vi "CheckNextState.vi"(0 "Car Wash IN":T1, 1 "Wash Options":bool[](array[boolean]), 2 "Current Step":i8, 3 "TimeHasElapsed?":bool) -> (7 "Car Wash OUT":T1, 8 "Next Step":i8)   [LabVIEW 2019]
uses:
  Controls/Car Wash Indicators.ctl
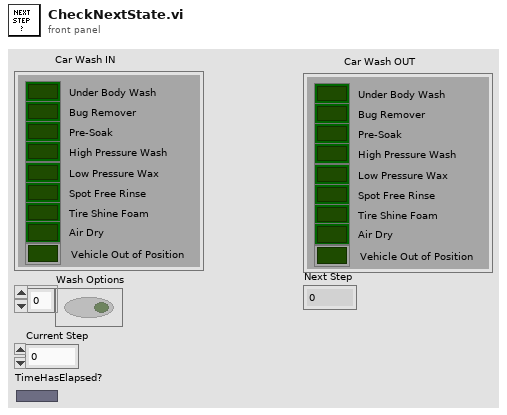
[diagram p1: front panel]
types:
  T1 = typedef "Car Wash Indicators.ctl" = cluster{"Under Body Wash":bool, "Bug Remover":bool, "Pre-Soak":bool, "High Pressure Wash":bool, "Low Pressure Wax":bool, "Spot Free Rinse":bool, "Tire Shine Foam":bool, "Air Dry":bool, "Vehicle Out of Position":bool}
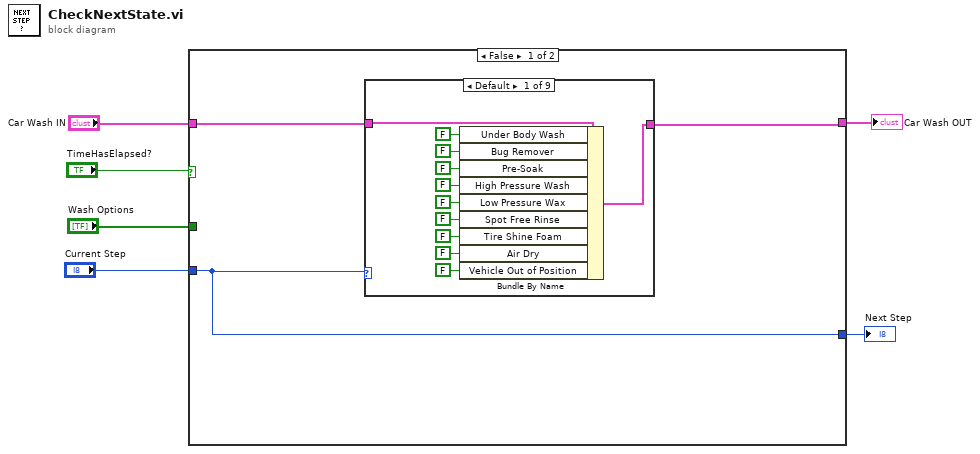
[diagram p0: block diagram]
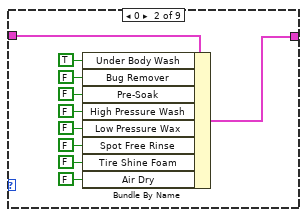
[diagram p2: hidden frame]
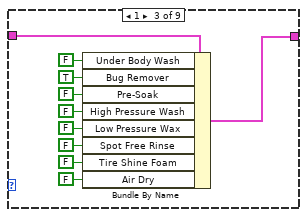
[diagram p3: hidden frame]
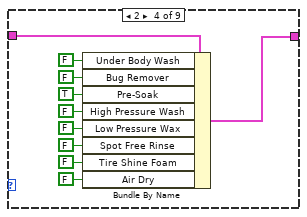
[diagram p4: hidden frame]
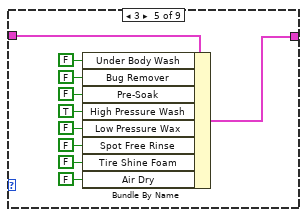
[diagram p5: hidden frame]
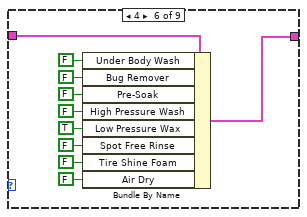
[diagram p6: hidden frame]
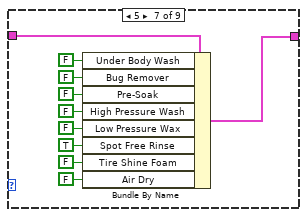
[diagram p7: hidden frame]
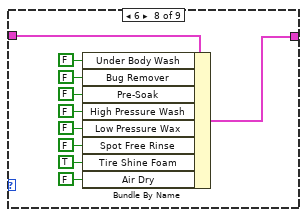
[diagram p8: hidden frame]
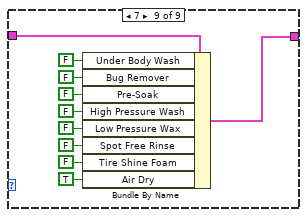
[diagram p9: hidden frame]
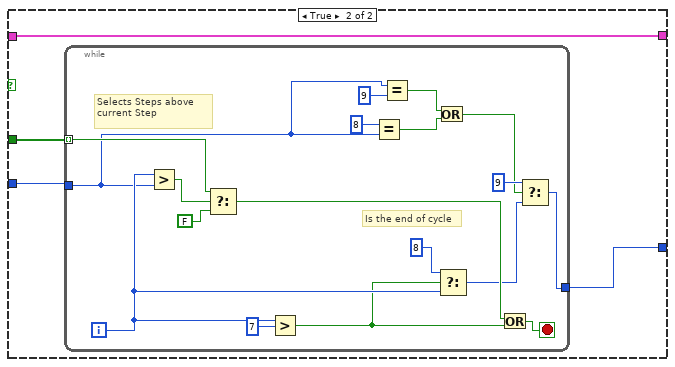
[diagram p10: hidden frame]
diagram:
  n1 = case shown="False" "TimeHasElapsed?" {
    tunnel: "Wash Options" -> [_ w104]
    tunnel: [w9 w103] -> w5
    tunnel: "Current Step" -> [w9 w102]
    tunnel: "Car Wash IN" -> [w8 w101]
    tunnel: [w7 w101] -> w1
    frame False {
      n2 = case shown="Default" w9 {
        tunnel: w8 -> [w11 w30 w40 w50 w60 w70 w80 w90 w100]
        tunnel: [w10 w21 w31 w41 w51 w61 w71 w81 w91] -> w7
        frame Default {
          n3 = Bundle By Name(cluster=w11, "Under Body Wash"=FALSE ("Vehicle Out of Position"), "Bug Remover"=FALSE, "Pre-Soak"=FALSE, "High Pressure Wash"=FALSE, "Low Pressure Wax"=FALSE, "Spot Free Rinse"=FALSE, "Tire Shine Foam"=FALSE, "Air Dry"=FALSE, "Vehicle Out of Position"=FALSE) -> (w10:T1)
        }
        frame 0 {
          n4 = Bundle By Name(cluster=w30, "Under Body Wash"=TRUE, "Bug Remover"=FALSE, "Pre-Soak"=FALSE, "High Pressure Wash"=FALSE, "Low Pressure Wax"=FALSE, "Spot Free Rinse"=FALSE, "Tire Shine Foam"=FALSE, "Air Dry"=FALSE) -> (w21:T1)
        }
        frame 1 {
          n5 = Bundle By Name(cluster=w40, "Under Body Wash"=FALSE, "Bug Remover"=TRUE, "Pre-Soak"=FALSE, "High Pressure Wash"=FALSE, "Low Pressure Wax"=FALSE, "Spot Free Rinse"=FALSE, "Tire Shine Foam"=FALSE, "Air Dry"=FALSE) -> (w31:T1)
        }
        frame 2 {
          n6 = Bundle By Name(cluster=w50, "Under Body Wash"=FALSE, "Bug Remover"=FALSE, "Pre-Soak"=TRUE, "High Pressure Wash"=FALSE, "Low Pressure Wax"=FALSE, "Spot Free Rinse"=FALSE, "Tire Shine Foam"=FALSE, "Air Dry"=FALSE) -> (w41:T1)
        }
        frame 3 {
          n7 = Bundle By Name(cluster=w60, "Under Body Wash"=FALSE, "Bug Remover"=FALSE, "Pre-Soak"=FALSE, "High Pressure Wash"=TRUE, "Low Pressure Wax"=FALSE, "Spot Free Rinse"=FALSE, "Tire Shine Foam"=FALSE, "Air Dry"=FALSE) -> (w51:T1)
        }
        frame 4 {
          n8 = Bundle By Name(cluster=w70, "Under Body Wash"=FALSE, "Bug Remover"=FALSE, "Pre-Soak"=FALSE, "High Pressure Wash"=FALSE, "Low Pressure Wax"=TRUE, "Spot Free Rinse"=FALSE, "Tire Shine Foam"=FALSE, "Air Dry"=FALSE) -> (w61:T1)
        }
        frame 5 {
          n9 = Bundle By Name(cluster=w80, "Under Body Wash"=FALSE, "Bug Remover"=FALSE, "Pre-Soak"=FALSE, "High Pressure Wash"=FALSE, "Low Pressure Wax"=FALSE, "Spot Free Rinse"=TRUE, "Tire Shine Foam"=FALSE, "Air Dry"=FALSE) -> (w71:T1)
        }
        frame 6 {
          n10 = Bundle By Name(cluster=w90, "Under Body Wash"=FALSE, "Bug Remover"=FALSE, "Pre-Soak"=FALSE, "High Pressure Wash"=FALSE, "Low Pressure Wax"=FALSE, "Spot Free Rinse"=FALSE, "Tire Shine Foam"=TRUE, "Air Dry"=FALSE) -> (w81:T1)
        }
        frame 7 {
          n11 = Bundle By Name(cluster=w100, "Under Body Wash"=FALSE, "Bug Remover"=FALSE, "Pre-Soak"=FALSE, "High Pressure Wash"=FALSE, "Low Pressure Wax"=FALSE, "Spot Free Rinse"=FALSE, "Tire Shine Foam"=FALSE, "Air Dry"=TRUE) -> (w91:T1)
        }
      }
    }
    frame True {
      n12 = while {
        tunnel: w104 -> [w122] mode=indexing
        tunnel: [w110] -> w103
        tunnel: w102 -> [w108]
        i -> [w116]
        stop <- w119 stop-if-true
        # "Selects Steps above\ncurrent Step"
        # "Is the end of cycle"
        n13 = Greater?(x=w116, y=w108) -> (0:w120:bool)
        n14 = Select(t=w122, s=w120, f=FALSE) -> (s? t:f=w117:bool)
        n15 = Greater?(x=w116, y=7) -> (0:w114:bool)
        n16 = Equal?(x=i8 8, y=w108) -> (x = y?=w106:bool)
        n17 = Equal?(x=w108, y=i8 9) -> (x = y?=w107:bool)
        n18 = Or(x=w107, y=w106) -> (x .or. y?=w105:bool)
        n19 = Select(t=8, s=w114, f=w116) -> (s? t:f=w112:i32)
        n20 = Or(x=w117, y=w114) -> (x .or. y?=w119:bool)
        n21 = Select(t=9, s=w105, f=w112) -> (s? t:f=w110:i32)
      }
    }
  }
  "Next Step" <- w5
  "Car Wash OUT" <- w1
